vi "Execute.vi"(6 "QD Text":string, 7 "QD Plugins Dir":path, 8 "error in (no error)":errorcluster, 9 "Shift?":bool, 10 "Focus":enum8{"FP", "BD"}(ring), 11 "VI Refnum":refnum<vi>) -> (0 "error out":errorcluster)   [LabVIEW 2019, in "Script.lvlib"]
doc: "Executes scripts shortcuts defined in the Quick Drop arguments.\n\nHelp: Ctrl-Space + \"?\" + Ctrl-S\n\nCreated by: Ryan Pacini"
uses:
  Script.lvlib
  Definitions.ctl
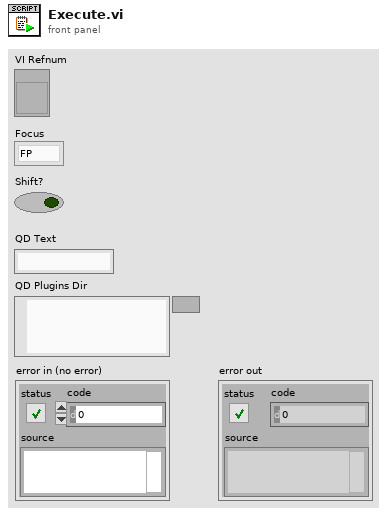
[diagram p1: front panel]
types:
  T1 = typedef "Script.lvlib/Definitions.ctl" = cluster{"plugins":cluster{"vi":path, "desc":string}[], "defaults":cluster{"uid":string, "name":string}[], "shortcuts":cluster{"shortcut":string, "uids":string[]}[], "defaults?":bool}
  T2 = enum16{"open", "replace", "create", "open or create", "replace or create", "replace or create with confirmation"}
  T3 = cluster{"name":string, "default":cluster{"uid":string, "name":string}}
  T4 = cluster{"name":string, "default":cluster{"uid":string, "name":string}}[]
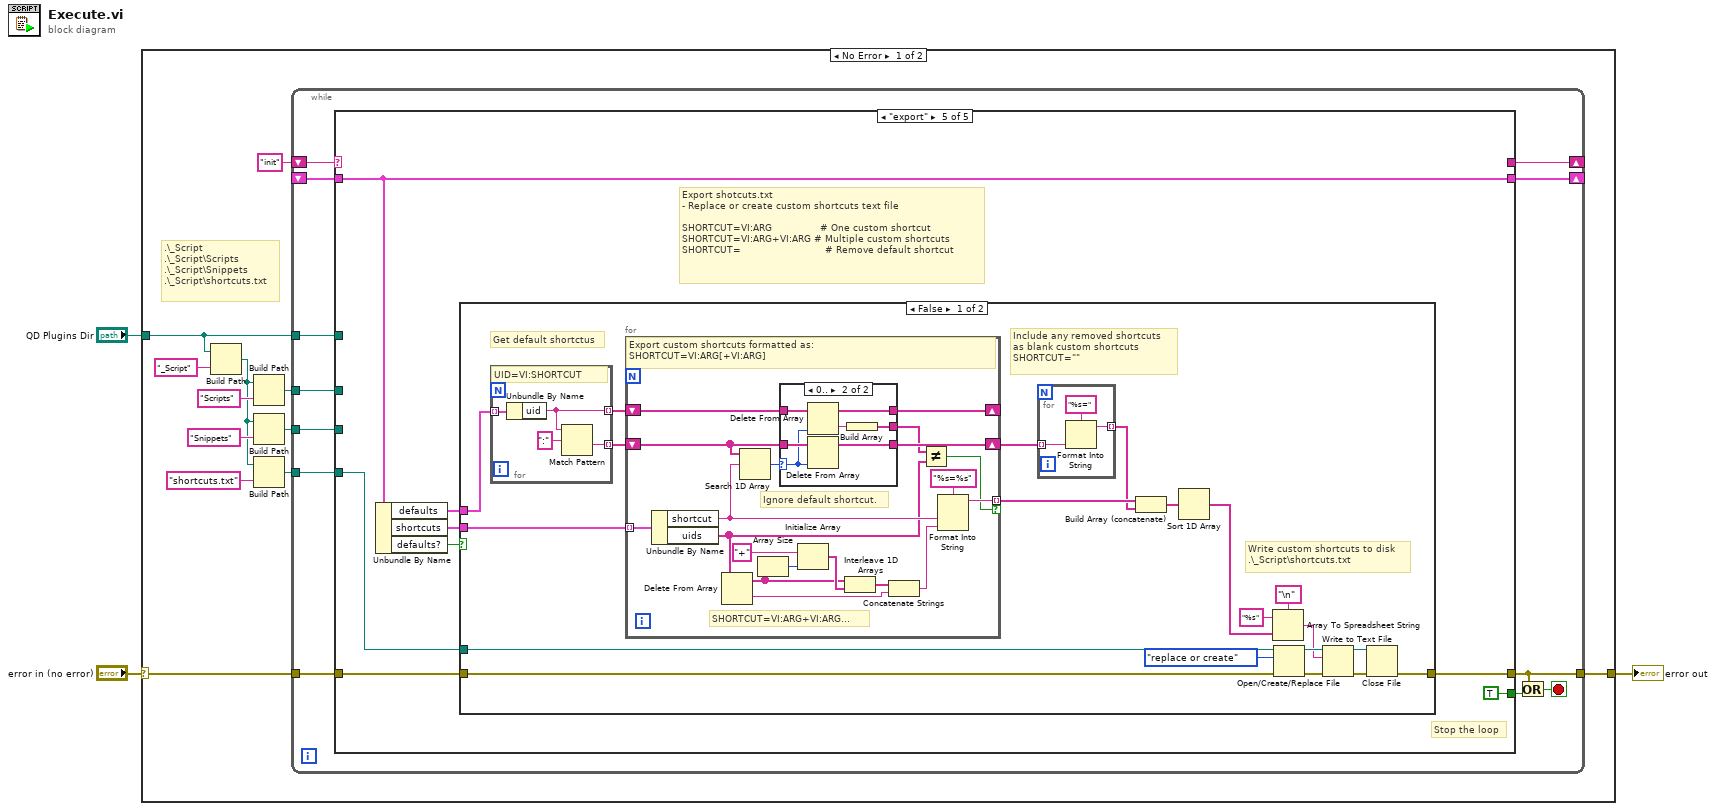
[diagram p0: block diagram]
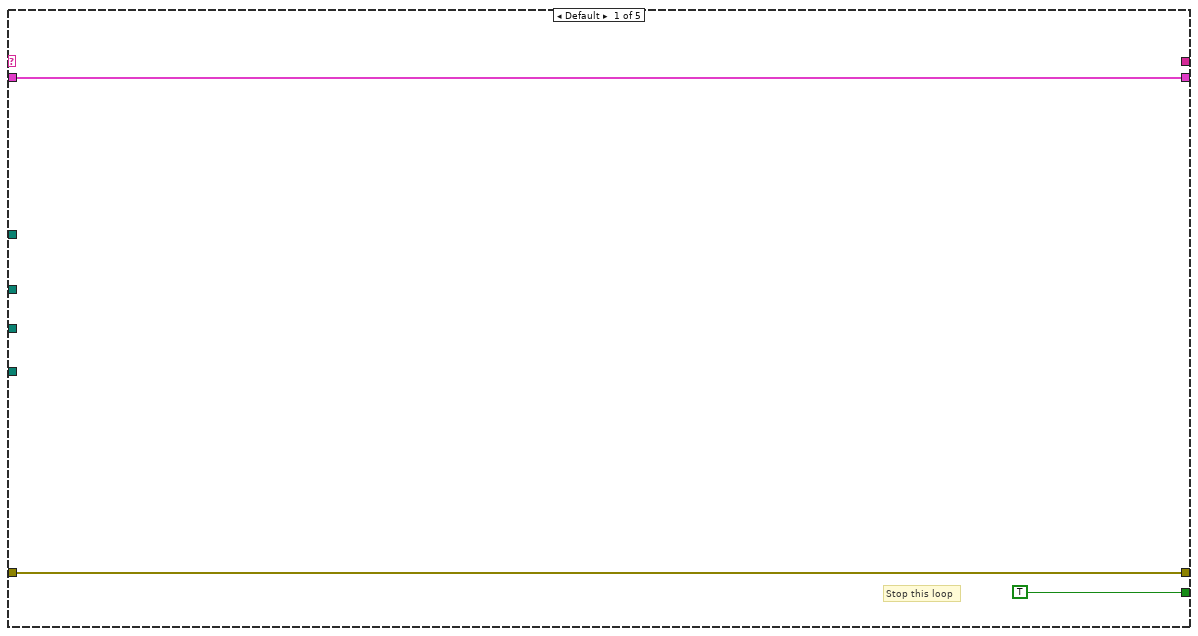
[diagram p2: hidden frame]
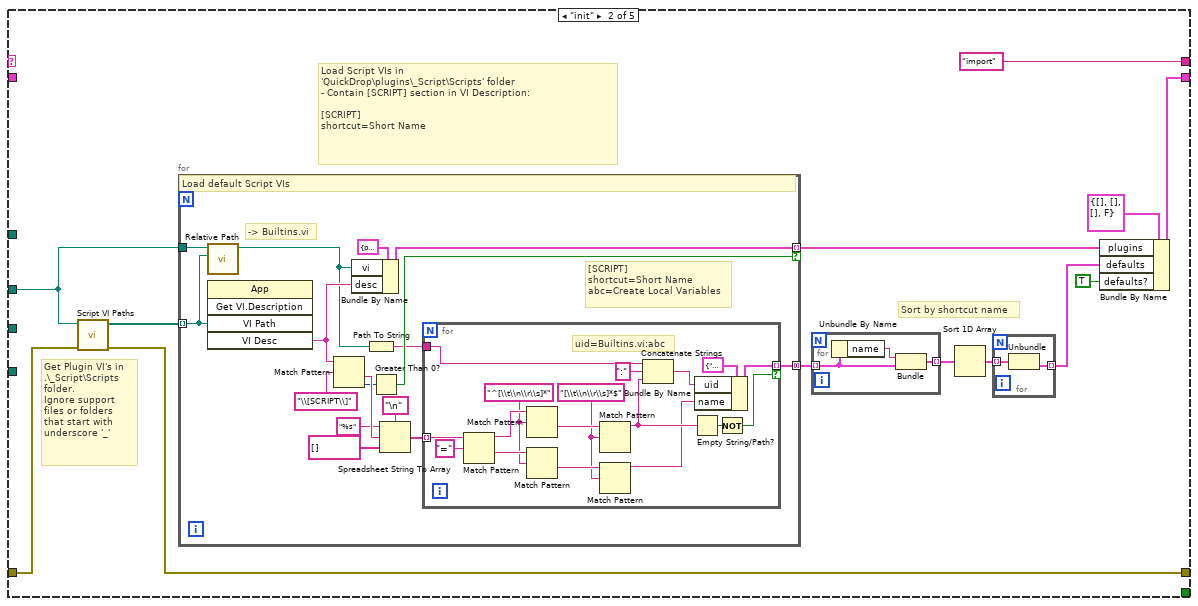
[diagram p3: hidden frame]
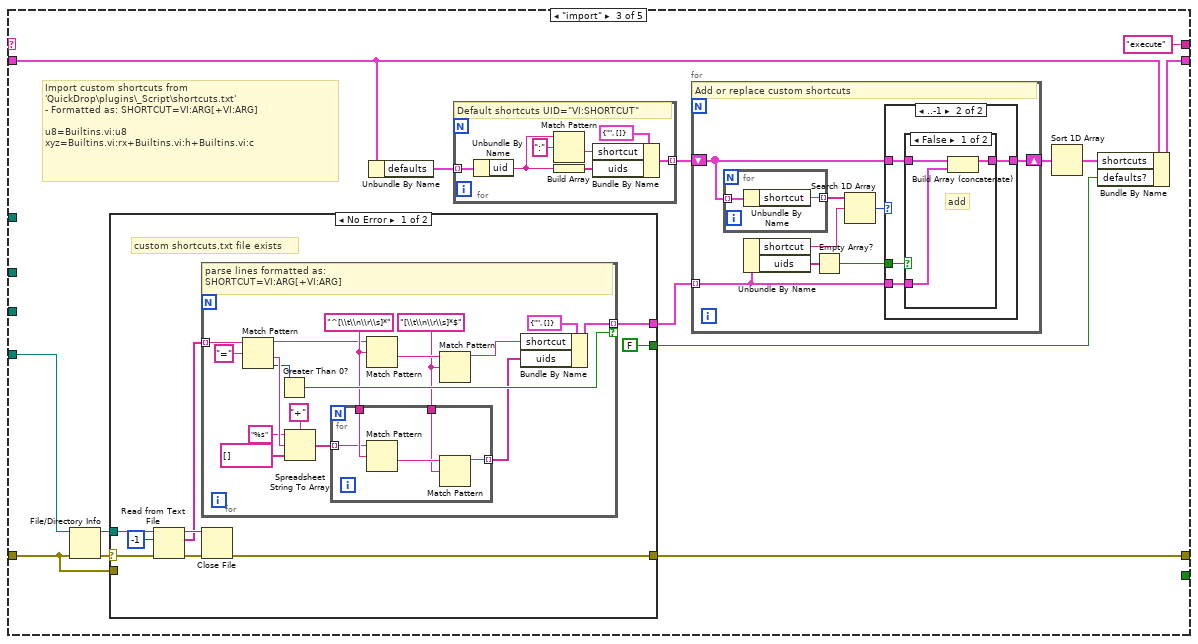
[diagram p4: hidden frame]
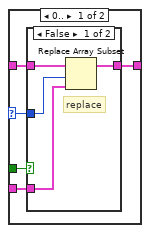
[diagram p5: hidden frame]
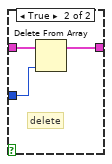
[diagram p6: hidden frame]
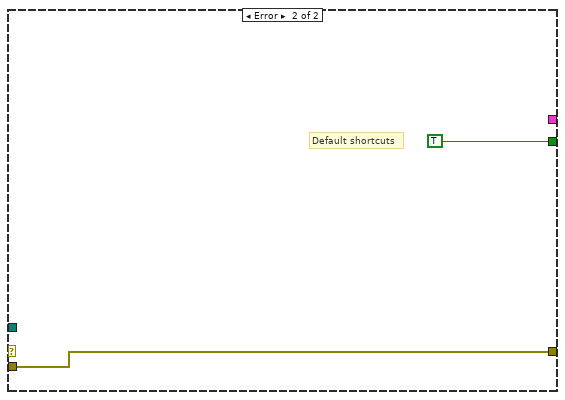
[diagram p8: hidden frame]
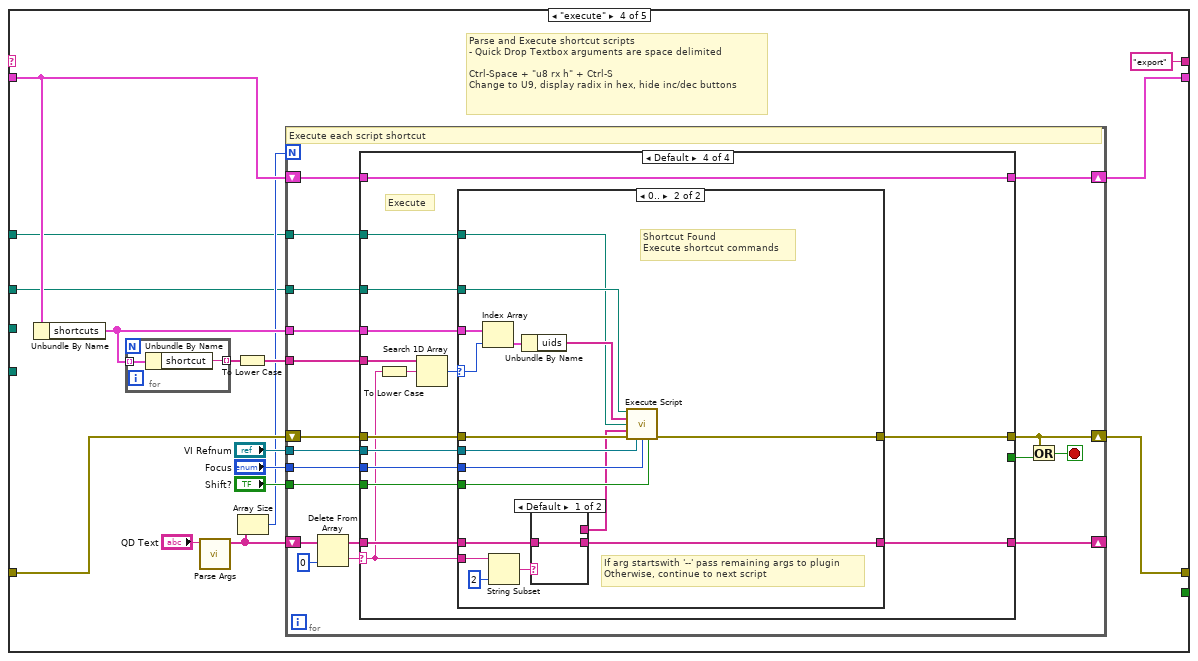
[diagram p9: hidden frame]
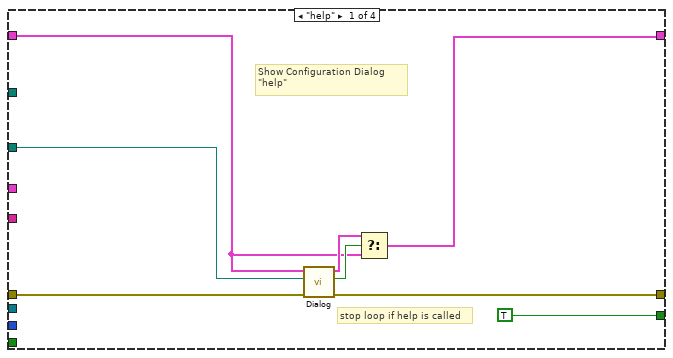
[diagram p10: hidden frame]
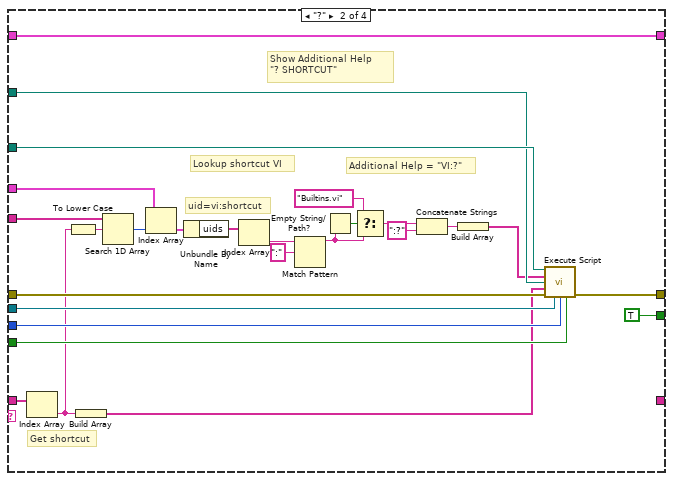
[diagram p11: hidden frame]
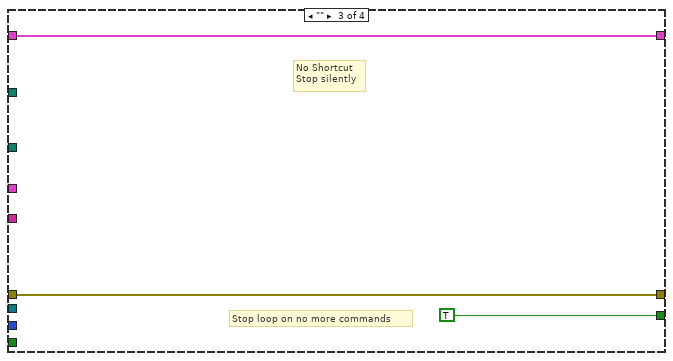
[diagram p12: hidden frame]
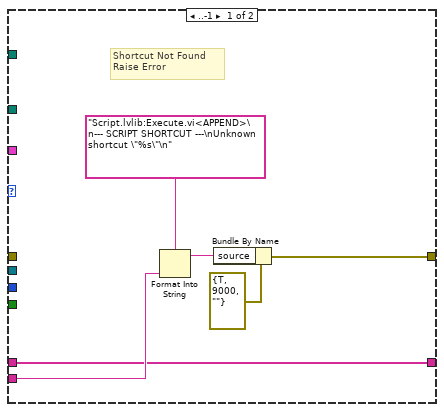
[diagram p13: hidden frame]
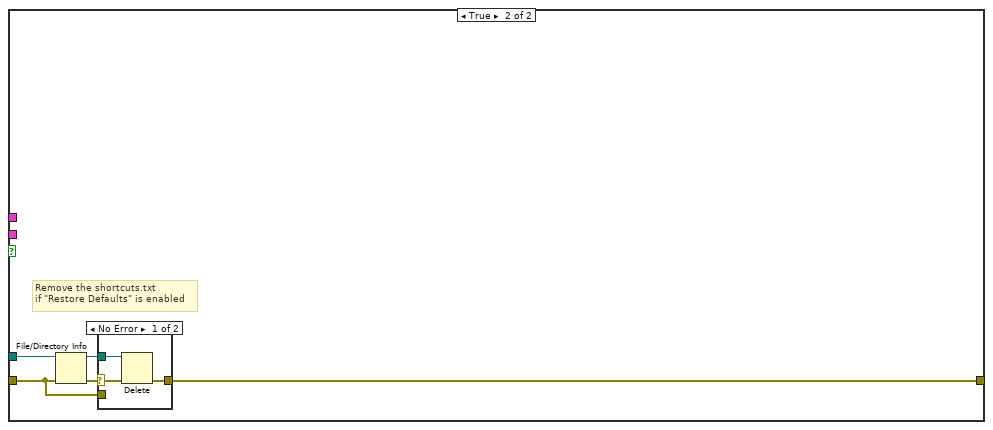
[diagram p16: hidden frame]
diagram:
  n1 = case shown="No Error" "error in (no error)" {
    selector: "error in (no error)" -> [w14 w352]
    tunnel: [w12 w352] -> w2
    tunnel: "QD Plugins Dir" -> [w10 _]
    frame No Error {
      # ".\\_Script\n.\\_Script\\Scripts\n.\\_Script\\Snippets\n.\\_Script\\shortcuts.txt"
      n2 = Build Path(base path=w10, name or relative path="_Script") -> (appended path=w4:path)
      n3 = Build Path(base path=w4, name or relative path="Scripts") -> (appended path=w8:path)
      n4 = Build Path(base path=w4, name or relative path="Snippets") -> (appended path=w5:path)
      n5 = Build Path(base path=w4, name or relative path="shortcuts.txt") -> (appended path=w9:path)
      n6 = while {
        tunnel: w14 -> [w27]
        shift-right: [w25] -> _
        shift-left: "init" -> [w26]
        shift-right: [w24] -> _
        shift-left: _ -> [w23]
        tunnel: [w22] -> w12
        tunnel: w10 -> [w19]
        tunnel: w9 -> [w18]
        tunnel: w8 -> [w17]
        tunnel: w5 -> [w16]
        stop <- w21 stop-if-true
        n7 = case shown="\"export\"" w26 {
          tunnel: w27 -> [w29 w35 w92 w181 w287]
          tunnel: [_ "import" "execute" "export" _] -> w25
          tunnel: [w30 w42 w90 w175 w284] -> w24
          tunnel: w23 -> [w30 _ w86 w171 w284]
          tunnel: [w29 w34 w95 w177 w286] -> w22
          tunnel: [TRUE _ _ _ TRUE] -> w20
          tunnel: w19 -> [_ _ _ w166 _]
          tunnel: w18 -> [_ _ w91 _ w285]
          tunnel: w17 -> [_ w31 _ w167 _]
          tunnel: w16 -> [_ _ _ _ _]
          frame Default {
            # "Stop this loop"
          }
          frame "init" {
            # "Load Script VIs in \n'QuickDrop\\plugins\\_Script\\Scripts' folder\n- Contain [SCRIPT] section in VI Description:\n\n[SCRIPT]\nshortcut=Short Name"
            # "Get Plugin VI's in \n.\\_Script\\Scripts \nfolder.\nIgnore support \nfiles or folders\nthat start with\nunderscore '_'"
            # "Sort by shortcut name"
            n8 = call "Script VI Paths.vi"("error in (no error)"=w35, "Directory"=w31) -> ("error out"=w34:errorcluster, "VI Paths"=w33:path[])  [unwired: 8 in]
            n9 = for {
              tunnel: w33 -> [w64] mode=indexing
              tunnel: [w63] -> w40 mode=indexing if=w62
              tunnel: w31 -> [w61]
              tunnel: [w60] -> w39 mode=concatenating
              # "-> Builtins.vi"
              # "[SCRIPT]\nshortcut=Short Name\nabc=Create Local Variables"
              # "Load default Script VIs"
              n10 = call "Relative Path.vi"("Child"=w64, "Parent"=w61) -> ("Child Relative Path"=w49:path)  [unwired: 9 in]
              n11 = invoke class="App" method="Get VI.Description"("VI Path"=w64) -> ("VI Desc"=w51:string)  [unwired: 4 in, 4 out]
              n12 = Match Pattern(string=w51, regular expression="\\[SCRIPT\\]") -> (after substring=w58:string, offset past match=w53:i32)  [unwired: 1 in, 2 out]
              n13 = Bundle By Name(cluster=cluster{"vi":path, "desc":string} {"vi"=path "", "desc"=""} ("plugin"), "vi"=w49, "desc"=w51) -> (w63:cluster{"vi":path, "desc":string})
              n14 = Path To String(path=w49) -> (string=w50:string)
              n15 = Greater Than 0?(x=w53) -> (x > 0?=w62:bool)
              n16 = Spreadsheet String To Array(delimiter (Tab)="\n", format string="%s", spreadsheet string=w58, array type (2D Dbl)=string[] []) -> (array=w54:string[])
              n17 = for {
                tunnel: w54 -> [w81] mode=indexing
                tunnel: [w66] -> w60 mode=indexing if=w72
                tunnel: w50 -> [w70]
                w74 = "[\\t\\n\\r\\s]*$" ("regular expression")
                w75 = "^[\\t\\n\\r\\s]*" ("regular expression")
                # "uid=Builtins.vi:abc"
                n18 = Match Pattern(string=w81, regular expression="=") -> (before substring=w78:string, after substring=w76:string)  [unwired: 1 in, 2 out]
                n19 = Match Pattern(string=w78, regular expression=w75) -> (after substring=w79:string)  [unwired: 1 in, 3 out]
                n20 = Match Pattern(string=w76, regular expression=w75) -> (after substring=w77:string)  [unwired: 1 in, 3 out]
                n21 = Match Pattern(string=w79, regular expression=w74) -> (before substring=w69:string)  [unwired: 1 in, 3 out]
                n22 = Match Pattern(string=w77, regular expression=w74) -> (before substring=w65:string)  [unwired: 1 in, 3 out]
                n23 = Concatenate Strings(w70, ":" ("string"), w69) -> (w67:string)
                n24 = Empty String/Path?(string/path=w69) -> (empty?=w73:bool)
                n25 = Bundle By Name(cluster=cluster{"uid":string, "name":string} {"uid"="", "name"=""} ("default"), "uid"=w67, "name"=w65) -> (w66:cluster{"uid":string, "name":string})
                n26 = Not(x=w73) -> (.not. x?=w72:bool)
              }
            }
            n27 = for {
              tunnel: w39 -> [w47] mode=indexing
              tunnel: [w46] -> w38 mode=indexing
              n28 = Unbundle By Name(w47) -> ("name"=w48:string)
              n29 = Bundle("name"=w48, "default"=w47) -> (w46:T3)  [unwired: 1 in]
            }
            n30 = Sort 1D Array(array=w38) -> (sorted array=w37:T4)
            n31 = for {
              tunnel: w37 -> [w45] mode=indexing
              tunnel: [w44] -> w36 mode=indexing
              n32 = Unbundle(w45) -> ("default"=w44:cluster{"uid":string, "name":string})  [unwired: 1 out]
            }
            n33 = Bundle By Name(cluster=T1 {"plugins"=[], "defaults"=[], "shortcuts"=[], "defaults?"=FALSE} ("data"), "plugins"=w40, "defaults"=w36, "defaults?"=TRUE) -> (w42:T1)
          }
          frame "import" {
            # "Import custom shortcuts from \n'QuickDrop\\plugins\\_Script\\shortcuts.txt'\n- Formatted as: SHORTCUT=VI:ARG[+VI:ARG]\n\nu8=Builtins.vi:u8\nxyz=Builtins.vi:rx+Builtins.vi:h+Builtins.vi:c"
            n34 = File/Directory Info(path=w91, error in=w92) -> (path out=w94:path, error out=w93:errorcluster)  [unwired: 5 out]
            n35 = case shown="No Error" w93 {
              selector: w93 -> [w140 _]
              tunnel: [w136 w165] -> w95
              tunnel: w94 -> [w141 _]
              tunnel: w92 -> [_ w165]
              tunnel: [FALSE TRUE] -> w87
              tunnel: [w133 _] -> w82
              frame No Error {
                # "custom shortcuts.txt file exists"
                n36 = Read from Text File(file (use dialog)=w141, count=-1, error in=w140) -> (refnum out=w137:refnum<file>, text=w134:string[], error out=w138:errorcluster)  [unwired: 1 in, 1 out]
                n37 = for {
                  tunnel: w134 -> [w158] mode=indexing
                  tunnel: [w149] -> w133 mode=indexing if=w151
                  w146 = "[\\t\\n\\r\\s]*$" ("regular expression")
                  w147 = "^[\\t\\n\\r\\s]*" ("regular expression")
                  # "parse lines formatted as:\nSHORTCUT=VI:ARG[+VI:ARG]"
                  n38 = Match Pattern(string=w158, regular expression="=") -> (before substring=w145:string, after substring=w156:string, offset past match=w152:i32)  [unwired: 1 in, 1 out]
                  n39 = Greater Than 0?(x=w152) -> (x > 0?=w151:bool)
                  n40 = Spreadsheet String To Array(delimiter (Tab)="+", format string="%s", spreadsheet string=w156, array type (2D Dbl)=string[] []) -> (array=w143:string[])
                  n41 = for {
                    tunnel: w147 -> [w162]
                    tunnel: w146 -> [w161]
                    tunnel: w143 -> [w160] mode=indexing
                    tunnel: [w159] -> w142 mode=indexing
                    n42 = Match Pattern(string=w160, regular expression=w162) -> (after substring=w163:string)  [unwired: 1 in, 3 out]
                    n43 = Match Pattern(string=w163, regular expression=w161) -> (before substring=w159:string)  [unwired: 1 in, 3 out]
                  }
                  n44 = Match Pattern(string=w145, regular expression=w147) -> (after substring=w148:string)  [unwired: 1 in, 3 out]
                  n45 = Match Pattern(string=w148, regular expression=w146) -> (before substring=w144:string)  [unwired: 1 in, 3 out]
                  n46 = Bundle By Name(cluster=cluster{"shortcut":string, "uids":string[]} {"shortcut"="", "uids"=[]} ("shortcut"), "shortcut"=w144, "uids"=w142) -> (w149:cluster{"shortcut":string, "uids":string[]})
                }
                n47 = Close File(refnum=w137, error in=w138) -> (error out=w136:errorcluster)  [unwired: 1 out]
              }
              frame Error {
                # "Default shortcuts"
              }
            }
            n48 = Unbundle By Name(w86) -> ("defaults"=w85:cluster{"uid":string, "name":string}[])
            n49 = for {
              tunnel: w85 -> [w131] mode=indexing
              tunnel: [w129] -> w84 mode=indexing
              # "Default shortcuts UID=\"VI:SHORTCUT\""
              n50 = Unbundle By Name(w131) -> ("uid"=w128:string)
              n51 = Match Pattern(string=w128, regular expression=":") -> (after substring=w126:string)  [unwired: 1 in, 3 out]
              n52 = Build Array(w128) -> (w130:string[])
              n53 = Bundle By Name(cluster=cluster{"shortcut":string, "uids":string[]} {"shortcut"="", "uids"=[]} ("shortcut"), "shortcut"=w126, "uids"=w130) -> (w129:cluster{"shortcut":string, "uids":string[]})
            }
            n54 = for {
              shift-right: [w100] -> w83
              shift-left: w84 -> [w103]
              tunnel: w82 -> [w99] mode=indexing
              # "Add or replace custom shortcuts"
              n55 = for {
                tunnel: w103 -> [w125] mode=indexing
                tunnel: [w124] -> w102 mode=indexing
                n56 = Unbundle By Name(w125) -> ("shortcut"=w124:string)
              }
              n57 = Unbundle By Name(w99) -> ("shortcut"=w101:string, "uids"=w97:string[])
              n58 = Empty Array?(array=w97) -> (empty?=w96:bool)
              n59 = Search 1D Array(1D array=w102, element=w101) -> (index of element=w98:i32)  [unwired: 1 in]
              n60 = case shown="..-1" w98 {
                selector: w98 -> [w105 _]
                tunnel: w103 -> [w108 w119]
                tunnel: [w107 w118] -> w100
                tunnel: w99 -> [w106 w117]
                tunnel: w96 -> [w104 w116]
                frame 0.. {
                  n61 = case shown="False" w104 {
                    tunnel: w108 -> [w112 w115]
                    tunnel: [w111 w113] -> w107
                    tunnel: w106 -> [w110 _]
                    tunnel: w105 -> [w109 w114]
                    frame False {
                      # "replace"
                      n62 = Replace Array Subset(array=w112, new element=w110, index=w109) -> (w111:cluster{"shortcut":string, "uids":string[]}[])
                    }
                    frame True {
                      # "delete"
                      n63 = Delete From Array(array=w115, index=w114) -> (array with subset deleted=w113:cluster{"shortcut":string, "uids":string[]}[])  [unwired: 1 in, 1 out]
                    }
                  }
                }
                frame ..-1 {
                  n64 = case shown="False" w116 {
                    tunnel: w119 -> [w122 w123]
                    tunnel: [w121 w123] -> w118
                    tunnel: w117 -> [w120 _]
                    frame False {
                      # "add"
                      n65 = Build Array (concatenate)(w122, w120) -> (w121:cluster{"shortcut":string, "uids":string[]}[])
                    }
                    frame True {
                      # "do not add"
                    }
                  }
                }
              }
            }
            n66 = Sort 1D Array(array=w83) -> (sorted array=w88:cluster{"shortcut":string, "uids":string[]}[])
            n67 = Bundle By Name(cluster=w86, "shortcuts"=w88, "defaults?"=w87) -> (w90:T1)
          }
          frame "execute" {
            # "Parse and Execute shortcut scripts\n- Quick Drop Textbox arguments are space delimited\n\nCtrl-Space + \"u8 rx h\" + Ctrl-S\nChange to U9, display radix in hex, hide inc/dec buttons"
            n68 = Unbundle By Name(w171) -> ("shortcuts"=w172:cluster{"shortcut":string, "uids":string[]}[])
            n69 = for {
              tunnel: w172 -> [w279] mode=indexing
              tunnel: [w278] -> w174 mode=indexing
              n70 = Unbundle By Name(w279) -> ("shortcut"=w278:string)
            }
            n71 = call "Parse Args.vi"("QD Text"="QD Text") -> ("args"=w168:string[])  [unwired: 10 in]
            n72 = To Lower Case(string=w174) -> (all lower case string=w173:string[])
            n73 = Array Size(array=w168) -> (size(s)=w169:i32)
            n74 = for {
              N: w169 -> [_]
              tunnel: w173 -> [w199]
              tunnel: w172 -> [w198]
              tunnel: "VI Refnum" -> [w196]
              tunnel: "Focus" -> [w195]
              tunnel: "Shift?" -> [w194]
              shift-right: [w190] -> w177
              shift-left: w181 -> [w197]
              shift-right: [w193] -> w175
              shift-left: w171 -> [w192]
              tunnel: w167 -> [w191]
              shift-right: [w184] -> _
              shift-left: w168 -> [w188]
              tunnel: w166 -> [w182]
              stop <- w186 stop-if-true
              # "Execute each script shortcut"
              n75 = Delete From Array(array=w188, index=0) -> (deleted portion=w183:string, array with subset deleted=w185:string[])  [unwired: 1 in]
              n76 = case shown="Default" w183 {
                selector: w183 -> [_ _ _ w240]
                tunnel: w199 -> [_ w226 _ w252]
                tunnel: w198 -> [_ w225 _ w250]
                tunnel: w197 -> [w207 w224 w236 w249]
                tunnel: w196 -> [_ w222 _ w248]
                tunnel: w195 -> [_ w221 _ w247]
                tunnel: w194 -> [_ w219 _ w246]
                tunnel: [w206 w223 w236 w245] -> w190
                tunnel: [w202 w234 w237 w244] -> w193
                tunnel: w192 -> [w203 w234 w237 w244]
                tunnel: w191 -> [w201 w220 _ w243]
                tunnel: [TRUE TRUE TRUE _] -> w189
                tunnel: w185 -> [_ w227 _ w242]
                tunnel: [_ _ _ w241] -> w184
                tunnel: w182 -> [_ w216 _ w238]
                frame "help" {
                  # "Show Configuration Dialog\n\"help\""
                  # "stop loop if help is called"
                  n77 = call "Dialog.vi"("error in (no error)"=w207, "Scripts Dir"=w201, "Definitions in"=w203) -> ("error out"=w206:errorcluster, "commit?"=w205:bool, "Definitions out"=w204:T1)  [unwired: 6 in]
                  n78 = Select(t=w204, s=w205, f=w203) -> (s? t:f=w202:T1)
                }
                frame "?" {
                  # "Additional Help = \"VI:?\""
                  # "Lookup shortcut VI"
                  # "uid=vi:shortcut"
                  # "Show Additional Help \n\"? SHORTCUT\""
                  # "Get shortcut"
                  n79 = Index Array(array=w227) -> (element=w218:string)  [unwired: 1 in]
                  n80 = To Lower Case(string=w218) -> (all lower case string=w233:string)
                  n81 = Build Array(w218) -> (w217:string[])
                  n82 = Search 1D Array(1D array=w226, element=w233) -> (index of element=w232:i32)  [unwired: 1 in]
                  n83 = Index Array(array=w225, index=w232) -> (element=w231:cluster{"shortcut":string, "uids":string[]})
                  n84 = Unbundle By Name(w231) -> ("uids"=w230:string[])
                  n85 = Index Array(array=w230) -> (element=w228:string)  [unwired: 1 in]
                  n86 = Match Pattern(string=w228, regular expression=":") -> (before substring=w214:string)  [unwired: 1 in, 3 out]
                  n87 = Empty String/Path?(string/path=w214) -> (empty?=w215:bool)
                  n88 = Select(t="Builtins.vi", s=w215, f=w214) -> (s? t:f=w211:string)
                  n89 = Concatenate Strings(w211, ":?" ("string")) -> (w209:string)
                  n90 = Build Array(w209) -> (w208:string[])
                  n91 = call "Execute Script.vi"("Scripts Dir"=w220, "uids"=w208, "QD Plugins Dir"=w216, "Arguments"=w217, "error in (no error)"=w224, "VI Refnum"=w222, "Focus"=w221, "Shift?"=w219) -> ("error out"=w223:errorcluster)  [unwired: 7 in]
                }
                frame "" {
                  # "No Shortcut\nStop silently"
                  # "Stop loop on no more commands"
                }
                frame Default {
                  # "Execute"
                  n92 = To Lower Case(string=w240) -> (all lower case string=w239:string)
                  n93 = Search 1D Array(1D array=w252, element=w239) -> (index of element=w251:i32)  [unwired: 1 in]
                  n94 = case shown="0.." w251 {
                    selector: w251 -> [_ w275]
                    tunnel: w250 -> [_ w274]
                    tunnel: w249 -> [_ w272]
                    tunnel: w248 -> [_ w265]
                    tunnel: w247 -> [_ w264]
                    tunnel: w246 -> [_ w263]
                    tunnel: [w257 w271] -> w245
                    tunnel: w243 -> [_ w260]
                    tunnel: w240 -> [w256 w269]
                    tunnel: w242 -> [w253 w267]
                    tunnel: [w253 w266] -> w241
                    tunnel: w238 -> [_ w259]
                    frame ..-1 {
                      # "Shortcut Not Found\nRaise Error"
                      n95 = Format Into String(format string="Script.lvlib:Execute.vi<APPEND>\n--- SCRIPT SHORTCUT ---\nUnknown shortcut \"%s\"\n" ("source"), w256) -> (resulting string=w254:string)  [unwired: 2 in, 1 out]
                      n96 = Bundle By Name(cluster=errorcluster {"status"=TRUE, "code"=9000, "source"=""} ("error IO"), "source"=w254) -> (w257:errorcluster)
                    }
                    frame 0.. {
                      # "Shortcut Found\nExecute shortcut commands"
                      # "If arg startswith '--' pass remaining args to plugin\nOtherwise, continue to next script"
                      n97 = Index Array(array=w274, index=w275) -> (element=w273:cluster{"shortcut":string, "uids":string[]})
                      n98 = String Subset(string=w269, length (rest)=2 ("length (rest)")) -> (substring=w268:string)  [unwired: 1 in]
                      n99 = Unbundle By Name(w273) -> ("uids"=w261:string[])
                      n100 = case shown="Default" w268 {
                        tunnel: w267 -> [w276 w277]
                        tunnel: [w276 _] -> w266
                        tunnel: [_ w277] -> w262
                        frame Default {
                        }
                        frame "--" {
                        }
                      }
                      n101 = call "Execute Script.vi"("Scripts Dir"=w260, "uids"=w261, "QD Plugins Dir"=w259, "Arguments"=w262, "error in (no error)"=w272, "VI Refnum"=w265, "Focus"=w264, "Shift?"=w263) -> ("error out"=w271:errorcluster)  [unwired: 7 in]
                    }
                  }
                }
              }
              n102 = Or(x=w190, y=w189) -> (x .or. y?=w186:bool)
            }
          }
          frame "export" {
            # "Export shotcuts.txt\n- Replace or create custom shortcuts text file\n\nSHORTCUT=VI:ARG                # One custom shortcut\nSHORTCUT=VI:ARG+VI:ARG # Multiple custom shortcuts\nSHORTCUT=                            # Remove default shortcut"
            # "Stop the loop"
            n103 = Unbundle By Name(w284) -> ("defaults"=w280:cluster{"uid":string, "name":string}[], "shortcuts"=w283:cluster{"shortcut":string, "uids":string[]}[], "defaults?"=w281:bool)
            n104 = case shown="False" w281 {
              tunnel: w287 -> [w307 w343]
              tunnel: [w297 w344] -> w286
              tunnel: w285 -> [w296 w347]
              tunnel: w283 -> [w295 _]
              tunnel: w280 -> [w294 _]
              frame False {
                # "Include any removed shortcuts\nas blank custom shortcuts\nSHORTCUT=\"\""
                # "Get default shortctus"
                # "Write custom shortcuts to disk\n.\\_Script\\shortcuts.txt"
                n105 = for {
                  tunnel: w294 -> [w314] mode=indexing
                  tunnel: [w312] -> w293 mode=indexing
                  tunnel: [w311] -> w292 mode=indexing
                  # "UID=VI:SHORTCUT"
                  n106 = Unbundle By Name(w314) -> ("uid"=w311:string)
                  n107 = Match Pattern(string=w311, regular expression=":") -> (after substring=w312:string)  [unwired: 1 in, 3 out]
                }
                n108 = for {
                  tunnel: [w333] -> w306 mode=indexing if=w324
                  tunnel: w295 -> [w332] mode=indexing
                  shift-right: [w316] -> w291
                  shift-left: w293 -> [w318]
                  shift-right: [w317] -> _
                  shift-left: w292 -> [w319]
                  # "SHORTCUT=VI:ARG+VI:ARG..."
                  # "Ignore default shortcut."
                  # "Export custom shortcuts formatted as:\nSHORTCUT=VI:ARG[+VI:ARG]"
                  n109 = Unbundle By Name(w332) -> ("shortcut"=w326:string, "uids"=w321:string[])
                  n110 = Delete From Array(array=w321) -> (deleted portion=w323:string, array with subset deleted=w320:string[])  [unwired: 2 in]
                  n111 = Search 1D Array(1D array=w318, element=w326) -> (index of element=w325:i32)  [unwired: 1 in]
                  n112 = Array Size(array=w320) -> (size(s)=w329:i32)
                  n113 = case shown="0.." w325 {
                    selector: w325 -> [_ w340]
                    tunnel: w319 -> [w335 w342]
                    tunnel: [_ w336] -> w315
                    tunnel: w318 -> [w334 w341]
                    tunnel: [w335 w339] -> w317
                    tunnel: [w334 w338] -> w316
                    frame ..-1 {
                    }
                    frame 0.. {
                      n114 = Delete From Array(array=w342, index=w340) -> (deleted portion=w337:string, array with subset deleted=w339:string[])  [unwired: 1 in]
                      n115 = Delete From Array(array=w341, index=w340) -> (array with subset deleted=w338:string[])  [unwired: 1 in, 1 out]
                      n116 = Build Array(w337) -> (w336:string[])
                    }
                  }
                  n117 = Initialize Array("+" ("delimiter (Tab)"), w329) -> (w322:string[])
                  n118 = Interleave 1D Arrays(w320, w322) -> (w328:string[])
                  n119 = Concatenate Strings(w328, w323) -> (w327:string)
                  n120 = Not Equal?(x=w315, y=w321) -> (x != y?=w324:bool)
                  n121 = Format Into String(format string="%s=%s", w326, w327) -> (resulting string=w333:string)  [unwired: 2 in, 1 out]
                }
                n122 = for {
                  tunnel: w291 -> [w309] mode=indexing
                  tunnel: [w308] -> w289 mode=indexing
                  n123 = Format Into String(format string="%s=", w309) -> (resulting string=w308:string)  [unwired: 2 in, 1 out]
                }
                n124 = Build Array (concatenate)(w306, w289) -> (w290:string[])
                n125 = Sort 1D Array(array=w290) -> (sorted array=w288:string[])
                n126 = Array To Spreadsheet String(delimiter (Tab)="\n", array=w288, 3:"%s" ("format string")) -> (spreadsheet string=w298:string)
                n127 = Open/Create/Replace File(file path (use dialog)=w296, error in=w307, operation (0:open)=T2."replace or create") -> (refnum out=w304:refnum<file>, error out=w305:errorcluster)  [unwired: 3 in, 1 out]
                n128 = Write to Text File(file (use dialog)=w304, text=w298, error in=w305) -> (refnum out=w303:refnum<file>, error out=w302:errorcluster)  [unwired: 1 in, 1 out]
                n129 = Close File(refnum=w303, error in=w302) -> (error out=w297:errorcluster)  [unwired: 1 out]
              }
              frame True {
                # "Remove the shortcuts.txt\nif \"Restore Defaults\" is enabled"
                n130 = File/Directory Info(path=w347, error in=w343) -> (path out=w345:path, error out=w346:errorcluster)  [unwired: 5 out]
                n131 = case shown="No Error" w346 {
                  selector: w346 -> [w350 _]
                  tunnel: w345 -> [w349 _]
                  tunnel: [w348 w351] -> w344
                  tunnel: w343 -> [_ w351]
                  frame No Error {
                    n132 = Delete(path (use dialog)=w349, error in=w350) -> (error out=w348:errorcluster)  [unwired: 3 in, 2 out]
                  }
                  frame Error {
                  }
                }
              }
            }
          }
        }
        n133 = Or(x=w22, y=w20) -> (x .or. y?=w21:bool)
      }
    }
    frame Error {
    }
  }
  "error out" <- w2
